vi "h.DETECTION.RemoveDetectionSetting.vi"(8 "error in":errorcluster, 10 "Detection Setting Index":u8, 11 "Connection ID":refnum<k5>) -> (0 "error out":errorcluster, 3 "Connection ID out":refnum<k5>)   [LabVIEW 2016, in "h.Library.lvlib"]
uses:
  h.Library.lvlib
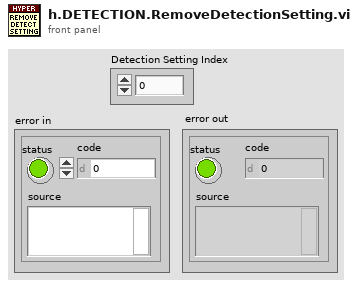
[diagram p1: front panel]
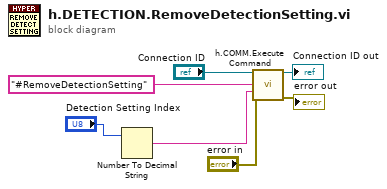
[diagram p0: block diagram]
diagram:
  n1 = Number To Decimal String(number="Detection Setting Index") -> (decimal integer string=w1:string)  [unwired: 1 in]
  n2 = call "h.COMM.Execute Command.vi"("Connection ID"="Connection ID", "Command"="#RemoveDetectionSetting", "Argument"=w1, "error in"="error in") -> ("Connection ID out"=→"Connection ID out":refnum<k5>, "error out"=→"error out":errorcluster)  [unwired: 4 in, 6 out]
